vi "3Reloj.vi"() -> ()   [LabVIEW 2016]
panel:
  out "Message":string
  out "Warning":bool
  out "Seconds":dbl
  out "Minutes":dbl
  out "Hours":dbl
  in  "Total Time in Seconds":dbl
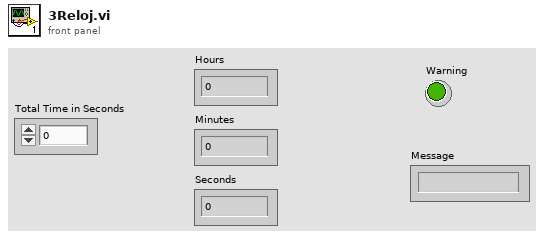
[diagram p1: front panel]
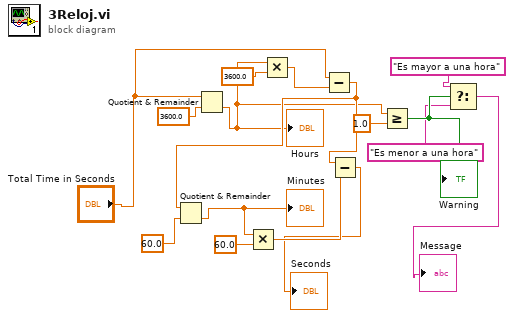
[diagram p0: block diagram]
diagram:
  n1 = Quotient & Remainder(x="Total Time in Seconds", y=3600.0) -> (floor(x/y)=w6:dbl)  [unwired: 1 out]
  "Hours" <- w6
  n2 = Multiply(x=w6, y=3600.0) -> (x*y=w11:dbl)
  n3 = Subtract(x="Total Time in Seconds", y=w11) -> (x-y=w8:dbl)
  n4 = Quotient & Remainder(x=w8, y=60.0) -> (floor(x/y)=w10:dbl)  [unwired: 1 out]
  "Minutes" <- w10
  n5 = Multiply(x=w10, y=60.0) -> (x*y=w9:dbl)
  n6 = Subtract(x=w8, y=w9) -> (x-y=→"Seconds":dbl)
  n7 = Greater Or Equal?(x=w6, y=1.0) -> (x >= y?=w4:bool)
  "Warning" <- w4
  n8 = Select(t="Es mayor a una hora", s=w4, f="Es menor a una hora") -> (s? t:f=→"Message":string)
